vi "Configure VI Server.vi"(8 "error in (no error)":errorcluster, 9 "Port (3363)":u32=3363, 10 "Enable? (true)":bool=TRUE, 11 "RT Management in":refnum<class "RT Management.lvclass">) -> (0 "error out":errorcluster, 3 "RT Management out":refnum<class "RT Management.lvclass">)   [LabVIEW 2015, in "RT Management.lvlib" / "RT Management.lvclass"]
doc: "Enables or disables VI Server on the target and sets the port number. By default, this method sets the VI and IP access tokens to \"+*\", allowing any VI or IP access. To configure these, use the Modify RT INI method following the Configure VI Server method. You can also set all four VI Server tokens via the Modify RT INI method as well."
uses:
  RT Management.lvclass
  controls/INI key.ctl
  RT Management.lvclass/RT Management.ctl
  Set Restart needed.vi
  RT Management.lvlib
panel:
  in  "Defer restart? (true)":bool=TRUE
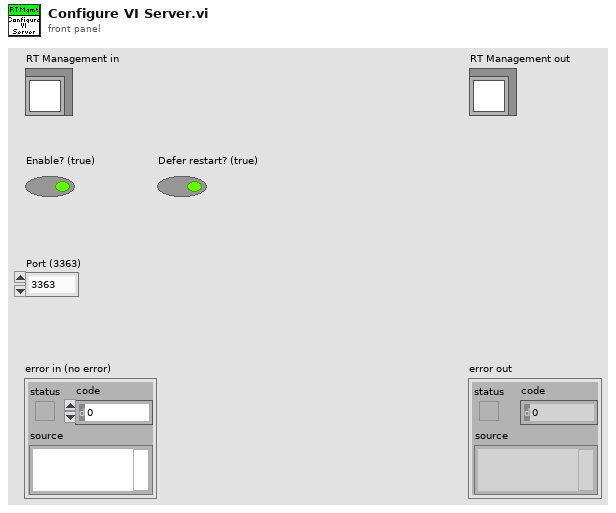
[diagram p1: front panel]
types:
  T1 = typedef "RT Management.lvlib/INI key.ctl" = cluster{"Section":string, "Key name":string, "Key value":string}
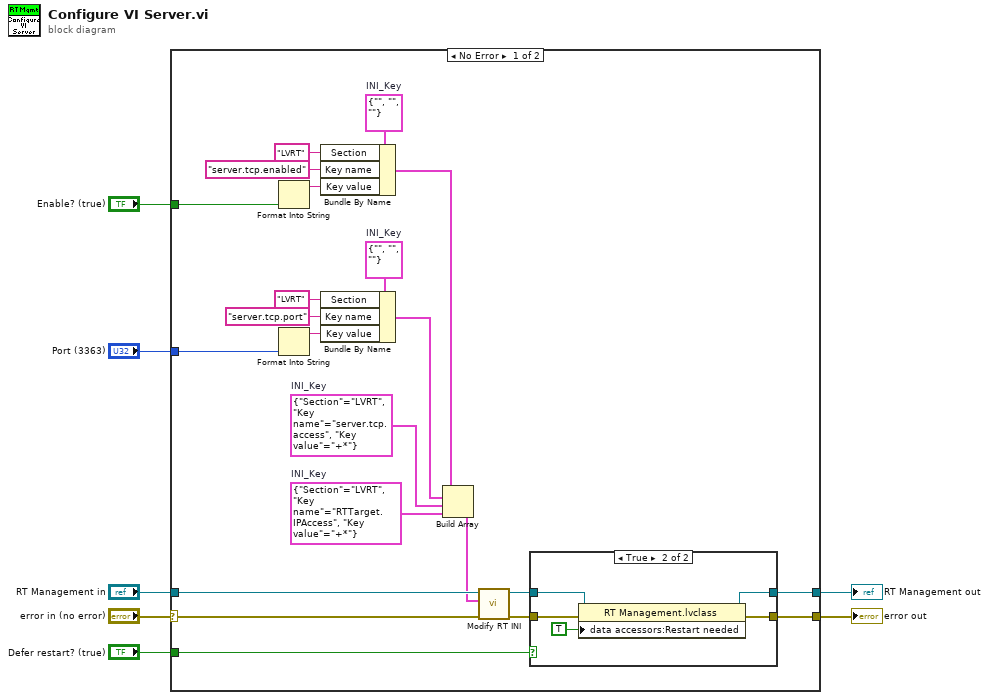
[diagram p0: block diagram]
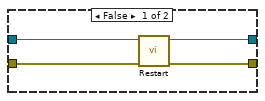
[diagram p2: hidden frame]
diagram:
  n1 = case shown="No Error" "error in (no error)" {
    selector: "error in (no error)" -> [w28 w40]
    tunnel: [w9 w40] -> w6
    tunnel: [w10 w39] -> w4
    tunnel: "RT Management in" -> [w29 w39]
    tunnel: "Enable? (true)" -> [w25 _]
    tunnel: "Port (3363)" -> [w18 _]
    tunnel: "Defer restart? (true)" -> [w8 _]
    frame No Error {
      w14 = T1 {"Section"="LVRT", "Key name"="RTTarget.IPAccess", "Key value"="+*"}  # INI_Key
      w15 = T1 {"Section"="LVRT", "Key name"="server.tcp.access", "Key value"="+*"}  # INI_Key
      w19 = T1 {"Section"="", "Key name"="", "Key value"=""}  # INI_Key
      w27 = T1 {"Section"="", "Key name"="", "Key value"=""}  # INI_Key
      n2 = Format Into String(w25) -> (resulting string=w24:string)  [unwired: 3 in, 1 out]
      n3 = Format Into String(w18) -> (resulting string=w21:string)  [unwired: 3 in, 1 out]
      n4 = Bundle By Name(cluster=w27, "Section"="LVRT", "Key name"="server.tcp.enabled", "Key value"=w24) -> (w17:T1)
      n5 = Bundle By Name(cluster=w19, "Section"="LVRT", "Key name"="server.tcp.port", "Key value"=w21) -> (w16:T1)
      n6 = Build Array(w17, w16, w15, w14) -> (w13:T1[])
      n7 = call "Modify RT INI.vi"("error in (no error)"=w28, "Keys to edit"=w13, "RT Management in"=w29) -> ("error out"=w12:errorcluster, "RT Management out"=w11:refnum<class "RT Management.lvclass">)  [unwired: 7 in]
      n8 = case shown="True" w8 {
        tunnel: w12 -> [w33 w38]
        tunnel: w11 -> [w32 w37]
        tunnel: [w31 w35] -> w10
        tunnel: [w30 w36] -> w9
        frame False {
          n9 = call "Restart.vi"("error in (no error)"=w33, "RT Management in"=w32) -> ("error out"=w30:errorcluster, "RT Management out"=w31:refnum<class "RT Management.lvclass">)  [unwired: 7 in]
        }
        frame True {
          n10 = property class="RT Management.lvclass"(reference=w37, error in=w38, "data accessors:Restart needed"=TRUE ("Restart needed")) -> (reference out=w35:refnum<class "RT Management.lvclass">, error out=w36:errorcluster)
        }
      }
    }
    frame Error {
    }
  }
  "error out" <- w6
  "RT Management out" <- w4
